vi "File_Set_MetaData.vi"(8 "error in (no error)":errorcluster, 10 "Meta Data":T1[](array[typedef]), 11 "File in":refnum<class "File.lvclass">) -> (0 "error out":errorcluster, 3 "File out":refnum<class "File.lvclass">)   [LabVIEW 2023, in "File.lvclass"]
doc: "Sets the metadata associated on the file level of the class."
uses:
  File.lvclass
  Meta Data.ctl
  File.lvclass/File.ctl
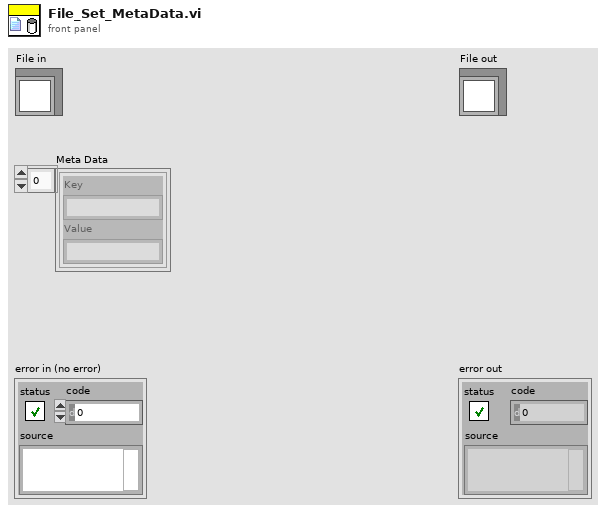
[diagram p1: front panel]
types:
  T1 = typedef "Meta Data.ctl" = cluster{"Key":string, "Value":string}
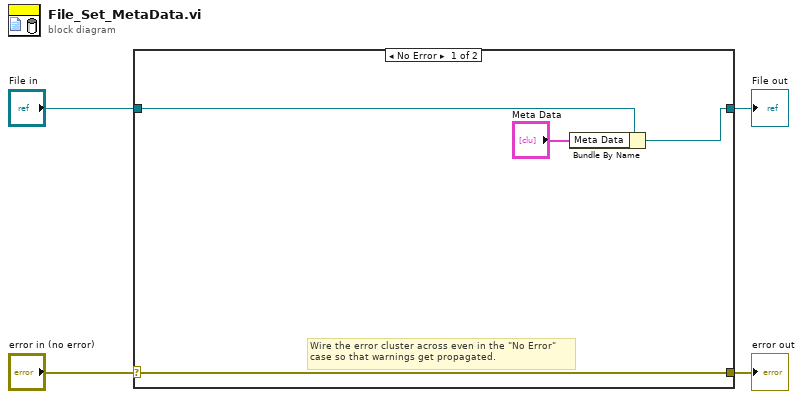
[diagram p0: block diagram]
diagram:
  n1 = case shown="No Error" "error in (no error)" {
    selector: "error in (no error)" -> [w8 w10]
    tunnel: [w8 w10] -> w3
    tunnel: [w6 w9] -> w1
    tunnel: "File in" -> [w7 w9]
    frame No Error {
      # "Wire the error cluster across even in the \"No Error\"\ncase so that warnings get propagated."
      n2 = Bundle By Name(cluster=w7, "Meta Data"="Meta Data") -> (w6:refnum<class "File.lvclass">)
    }
    frame Error {
    }
  }
  "error out" <- w3
  "File out" <- w1
